vi "FPGASteeringValidateWithTime.vi"() -> ()   [LabVIEW 2016]
uses:
  <vilib>/Platform/TimedLoop/XDataNode/timing_clust.ctl
  <vilib>/Platform/TimedLoop/XDataNode/nitl_modes.ctl
  <vilib>/Platform/TimedLoop/XDataNode/wakeup.ctl
  <vilib>/rvi/Emulation/niFpgaGetClockAttributes.vi
  <vilib>/rvi/Emulation/niFpgaSctlEmulationGetInTimedLoop.vi
  <vilib>/rvi/Emulation/niFpgaEmulationReportErrorSimple.vi
  <vilib>/rvi/Emulation/niFpgaProcessEmulError.vi
  <vilib>/rvi/Emulation/niFpgaCriticalErrorInLSC.vi
  <vilib>/rvi/eio/common/nirviEmuTemplateMethod_errors.vi
  <vilib>/eio/EIONode/EIONode.xnode
  <vilib>/Platform/TimedLoop/XDataNode/XDataNode.xnode
  <vilib>/Platform/TimedLoop/XDataNode/XDNodeRunTimeDep.lvlib
panel:
  in  "Front Panel Duty Cycle":sgl
  in  "Front Panel Direction":bool
  in  "Freq":u32=400000
  in  "Stop direction switch":bool
  in  "Direction":bool
  out "Position":i64
  in  "Stop encoder":bool
  in  "Reset counter":bool
  out "Steering angle(deg)":sgl
  out "Duty cycle (steering)":sgl
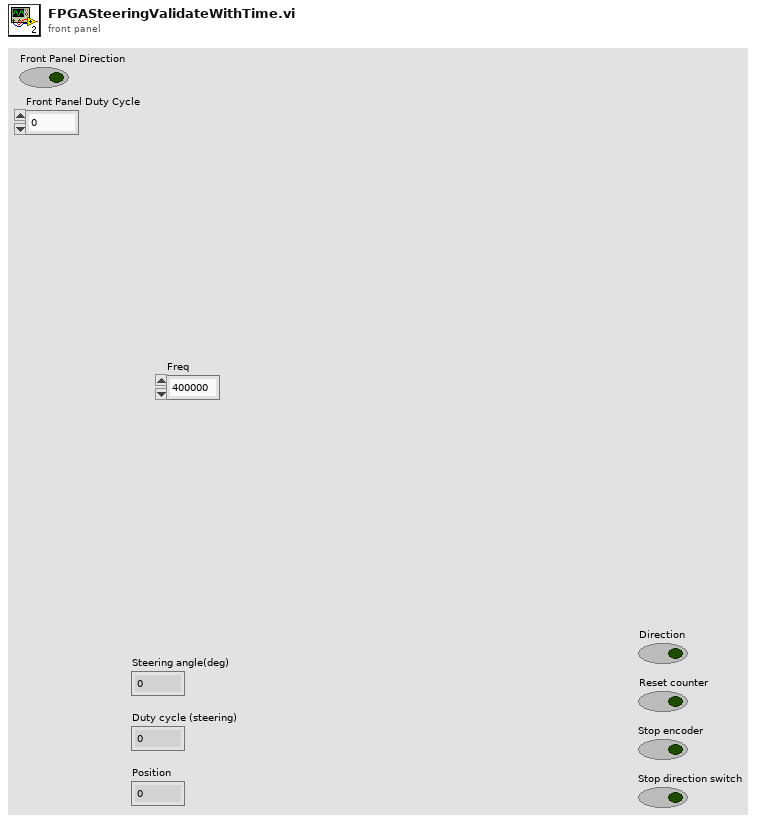
[diagram p1: front panel]
types:
  T1 = typedef "XDNodeRunTimeDep.lvlib/timing_clust.ctl" = cluster{"Expected End [f-1]":u64, "Actual End [f-1]":u64, "Finished Late? [f-1]":bool, "Expected End [i-1]":u64, "Actual End [i-1]":u64, "Finished Late? [i-1]":bool, "Expected Start [i]":u64, "Actual Start [i]":u64, "Expected Start [f]":u64, "Actual Start [f]":u64, "Source Name":string, "Structure Name":string, "Period":i64, "Deadline":i64, "Offset":i64, "Start":i64, "Priority":i32, "Timeout":i32, "Mode":T2, "Wakeup Reason":T3, "Error":errorcluster, "Source Type":string, "Secondary Source Type":string, "Global End Time":u64, "Global Start Time":u64, "Frame Duration":u64, "Iteration Duration":u64, "Assigned CPU":i32, "I/O Scan Engine Mode":u32}
  T2 = typedef "XDNodeRunTimeDep.lvlib/nitl_modes.ctl" = enum32{"No Change", "Process missed periods, maintain original phase", "Discard missed periods, maintain original phase", "Process missed periods, ignore original phase", "Discard missed periods, ignore original phase"}
  T3 = typedef "XDNodeRunTimeDep.lvlib/wakeup.ctl" = enum32{"Normal", "Aborted", "Asynchronous wakeup", "Timing source error", "Timed loop error", "Timeout"}
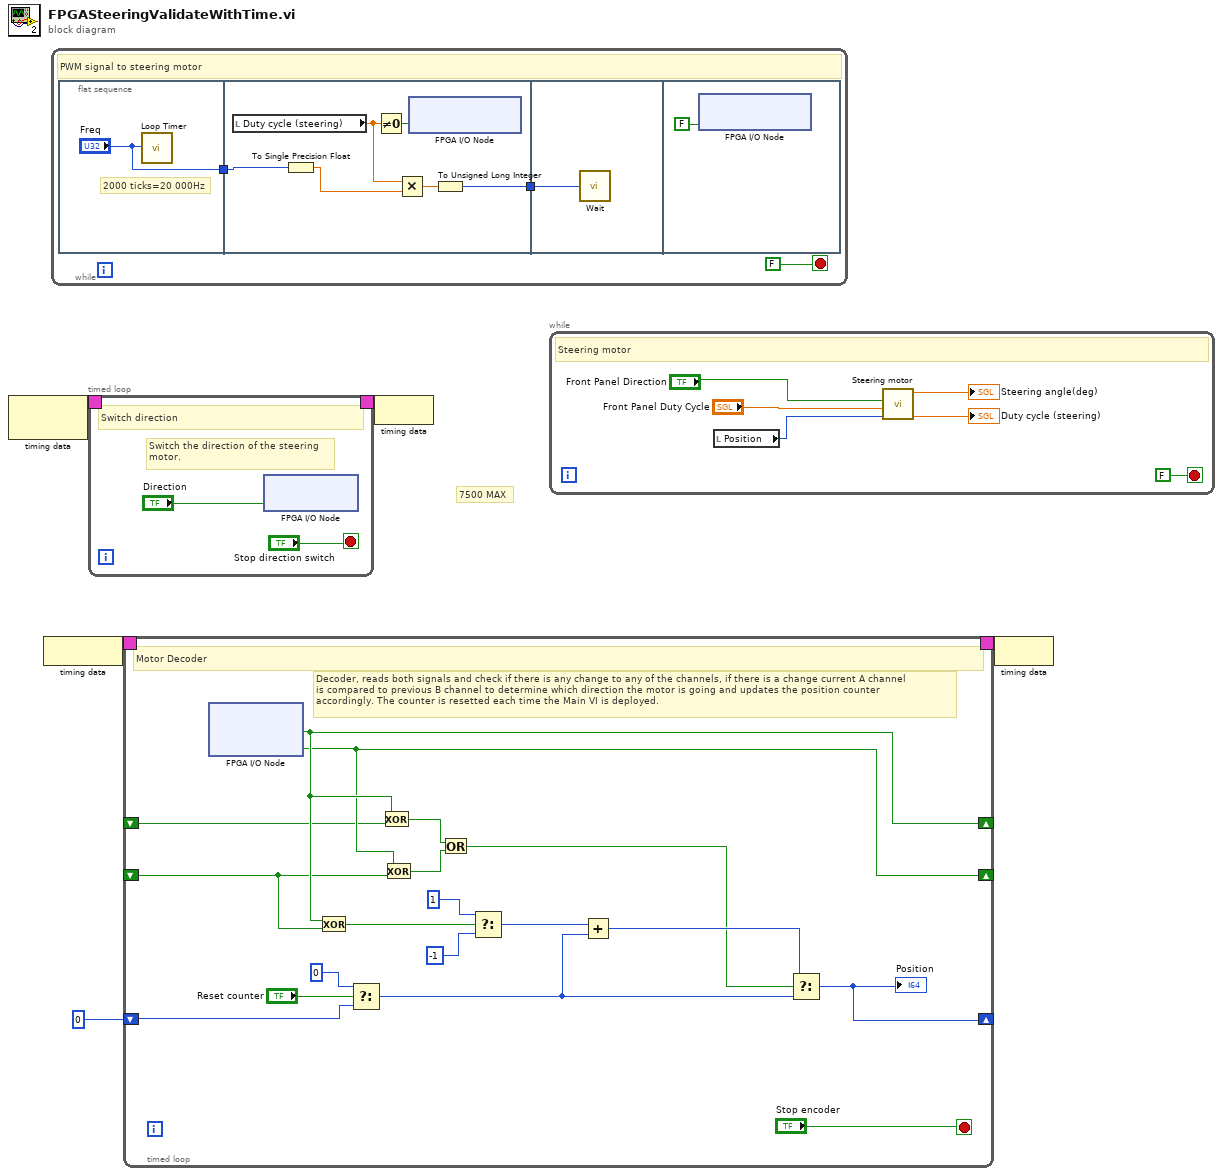
[diagram p0: block diagram]
diagram:
  # "7500 MAX"
  n1 = node-c288() -> (w5:T1)  [unwired: 1 in]
  n2 = node-c288() -> (w3:T1)
  n3 = while {
    stop <- FALSE stop-if-true
    # "PWM signal to steering motor"
    n4 = flat-sequence {
      tunnel: ["Freq"] -> w6
      tunnel: [w14] -> w8
      tunnel: w6 -> [w11]
      tunnel: w8 -> [w16]
      frame #0 {
        # "2000 ticks=20 000Hz"
        n5 = call "Loop Timer"("Count(Ticks)"="Freq") -> ()  [unwired: 1 out]
      }
      frame #1 {
        n6 = local read "Duty cycle (steering)"() -> (w12:sgl)
        n7 = To Single Precision Float(number=w11) -> (single precision float=w10:sgl)
        n8 = Not Equal To 0?(x=w12) -> (x != 0?=w13:bool)
        n9 = Multiply(x=w12, y=w10) -> (x*y=w15:sgl)
        n10 = xnode "FPGA I/O Node"("PWM/PWM0"=w13) -> ()  [unwired: 1 in, 1 out]
        n11 = To Unsigned Long Integer(number=w15) -> (unsigned 32bit integer=w14:u32)
      }
      frame #2 {
        n12 = call "Wait"("Count(Ticks)"=w16) -> ()  [unwired: 1 out]
      }
      frame #3 {
        n13 = xnode "FPGA I/O Node"("PWM/PWM0"=FALSE ("PWM/PWM8")) -> ()  [unwired: 1 in, 1 out]
      }
    }
  }
  n14 = timed-loop {
    timing: w5 -> [_]
    timing-out: [_] -> w4
    stop <- "Stop direction switch" stop-if-true
    # "Switch the direction of the steering\nmotor."
    # "Switch direction"
    n15 = xnode "FPGA I/O Node"("DIO/DIO2"="Direction") -> ()  [unwired: 1 in, 1 out]
  }
  n16 = timed-loop {
    shift-right: [w32] -> _
    shift-left: i64 0 ("t") -> [w23]
    shift-right: [w29] -> _
    shift-left: _ -> [w27]
    shift-right: [w28] -> _
    shift-left: _ -> [w26]
    timing: w3 -> [_]
    timing-out: [_] -> w2
    stop <- "Stop encoder" stop-if-true
    # "Decoder, reads both signals and check if there is any change to any of the channels, if there is a change current A channel\nis compared to previous B channel to determine which direction the motor is going and updates the position counter\naccordingly. The counter is resetted each time the Main VI is deployed."
    # "Motor Decoder"
    n17 = xnode "FPGA I/O Node"() -> ("DIO/DIO0"=w29:bool, "DIO/DIO1"=w28:bool)  [unwired: 2 in, 2 out]
    n18 = Exclusive Or(1:w26, 2:w29) -> (0:w25:bool)
    n19 = Select(t=i64 0, s="Reset counter", f=w23) -> (s? t:f=w31:i64)
    n20 = Exclusive Or(1:w27, 2:w29) -> (0:w39:bool)
    n21 = Exclusive Or(1:w26, 2:w28) -> (0:w38:bool)
    n22 = Or(x=w39, y=w38) -> (x .or. y?=w24:bool)
    n23 = Select(t=i64 1, s=w25, f=i64 -1) -> (s? t:f=w34:i64)
    n24 = Add(x=w34, y=w31) -> (x+y=w33:i64)
    n25 = Select(t=w33, s=w24, f=w31) -> (s? t:f=w32:i64)
    "Position" <- w32
  }
  n26 = node-c288(w4) -> ()
  n27 = while {
    stop <- FALSE stop-if-true
    # "Steering motor"
    n28 = local read "Position"() -> (w46:i64)
    n29 = call "Steering motor.vi"("Steering position (in pulses)"=w46, "Duty Cycle in"="Front Panel Duty Cycle", "Switch direction"="Front Panel Direction") -> ("Duty Cycle out"=→"Duty cycle (steering)":sgl, "Steering angle(deg)"=→"Steering angle(deg)":sgl)  [unwired: 7 in]
  }
  n30 = node-c288(w2) -> ()
